vi "controller.vi"(2 "P2X":dbl, 3 "P1X":dbl, 4 "ForceY":dbl, 5 "ForceX":dbl, 6 "dispY":dbl, 7 "dispX":dbl, 8 "Dc":dbl[](array[numeric])=[0.0, 0.0], 9 "Cc":dbl[](array[numeric])=[1.0, 0.0], 10 "Bc":dbl[](array[numeric])=[1.0, 1.0], 11 "Ac":dbl[](array[numeric])=[0.5, 1.0]) -> (0 "VALVECMDY":dbl, 1 "VALVECMDX":dbl)   [LabVIEW 2023]
uses:
  <vilib>/Analysis/baseanly.llb/A x Vector.vi
  <vilib>/Analysis/NI_AALBase.lvlib
  <vilib>/Analysis/NI_AALBLAS.lvlib
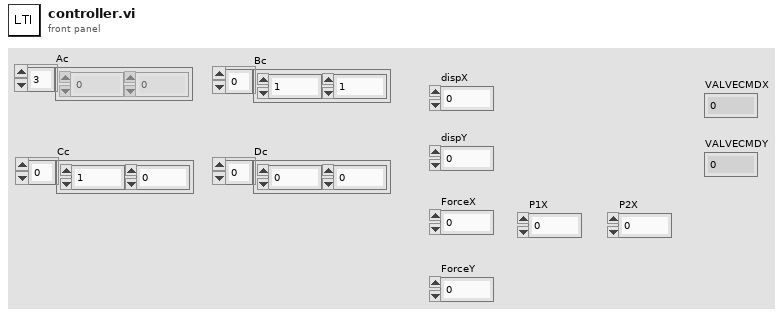
[diagram p1: front panel]
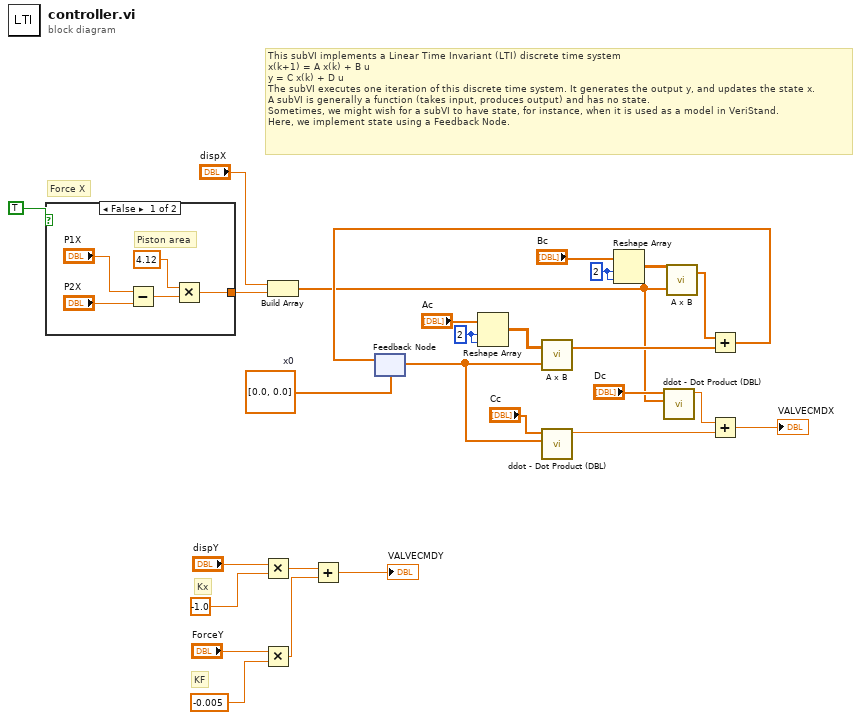
[diagram p0: block diagram]
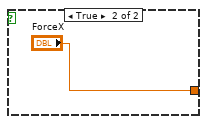
[diagram p2: hidden frame]
diagram:
  w4 = 2 ("dimension size")
  w5 = 2 ("dimension size")
  w27 = dbl[] [0.0, 0.0]  # x0
  # "KF"
  # "Kx"
  # "Force X"
  # "This subVI implements a Linear Time Invariant (LTI) discrete time system\nx(k+1) = A x(k) + B u\ny = C x(k) + D u\nThe subVI executes one iteration of this discrete time system. It generates the output y, and updates the state x.\nA subVI is generally a function (takes input, produces output) and has no state.\nSometimes, we might wish for a subVI to have state, for instance, when it is used as a model in VeriStand.\nHere, we implement state using a Feedback Node."
  n1 = case shown="False" TRUE {
    tunnel: [w28 "ForceX"] -> w15
    frame False {
      # "Piston area"
      n2 = Subtract(x="P1X", y="P2X") -> (x-y=w32:dbl)
      n3 = Multiply(x=4.12, y=w32) -> (x*y=w28:dbl)
    }
    frame True {
    }
  }
  n4 = Multiply(x="dispY", y=-1.0) -> (x*y=w10:dbl)
  n5 = Multiply(x="ForceY", y=-0.005) -> (x*y=w9:dbl)
  n6 = Build Array("dispX", w15) -> (w17:dbl[])
  n7 = Add(x=w10, y=w9) -> (x+y=→"VALVECMDY":dbl)
  n8 = feedback #1(w27) -> (w24:dbl[])
  n9 = Reshape Array("Ac", w5, w5) -> (w2:dbl[][])
  n10 = call-poly <vilib>:"A x B.vi"("Vector"=w24, "A"=w2) -> ("A x Vector"=w26:dbl[])  [unwired: 1 out]
  n11 = call <vilib>:"ddot - Dot Product (DBL).vi"("y"=w24, "x"="Cc") -> ("ddot"=w22:dbl)  [unwired: 8 in, 1 out]
  n12 = Reshape Array("Bc", w4, w4) -> (w1:dbl[][])
  n13 = call <vilib>:"ddot - Dot Product (DBL).vi"("y"=w17, "x"="Dc") -> ("ddot"=w19:dbl)  [unwired: 8 in, 1 out]
  n14 = call-poly <vilib>:"A x B.vi"("Vector"=w17, "A"=w1) -> ("A x Vector"=w21:dbl[])  [unwired: 1 out]
  n15 = Add(x=w21, y=w26) -> (x+y=w25:dbl[])
  n16 = feedback-in #1(w25) -> ()
  n17 = Add(x=w19, y=w22) -> (x+y=→"VALVECMDX":dbl)
